vi "FTW-TransferClient-Cancel.vi"(0 "Transfer Client":refnum<k24>, 11 "error in":errorcluster) -> (4 "Transfer Client out":refnum<k24>, 15 "error out":errorcluster)   [LabVIEW 2015]
panel:
  # "Inputs"
  # "Outputs"
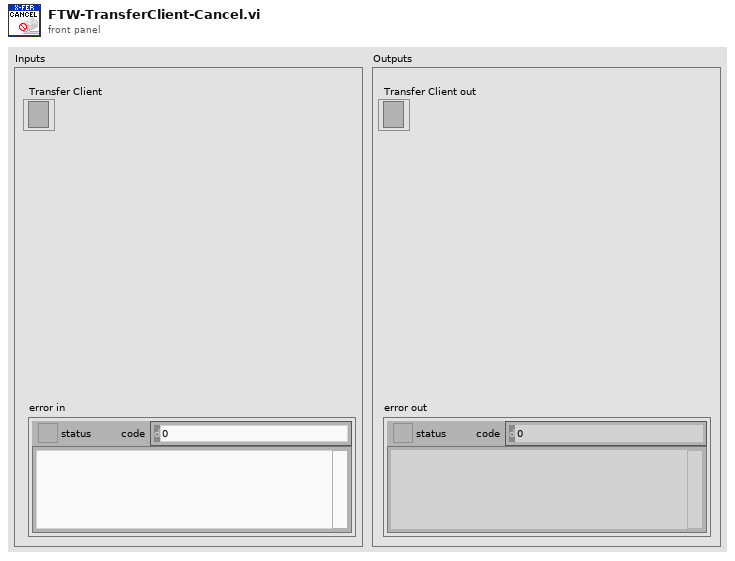
[diagram p1: front panel]
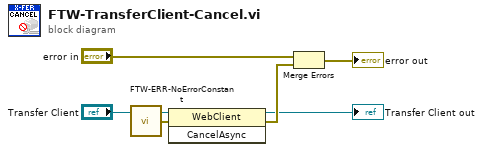
[diagram p0: block diagram]
diagram:
  n1 = call "FTW-ERR-NoErrorConstant.vi"() -> ("no error"=w1:errorcluster)
  n2 = invoke class="WebClient" method="CancelAsync"(reference="Transfer Client", error in=w1) -> (reference out=→"Transfer Client out":refnum<k24>, error out=w6:errorcluster)  [unwired: 1 in, 1 out]
  n3 = Merge Errors("error in", w6) -> (→"error out":errorcluster)
